vi "test4-EndNodeHandlesErrorForNotAllowedMessages.vi"(8 "error in (no error)":errorcluster, 11 "TestCase in":refnum<class "testcase-CSMChainMode.lvclass">) -> (0 "error out":errorcluster, 3 "TestCase out":refnum<class "testcase-CSMChainMode.lvclass">)   [LabVIEW 2017, in "testcase-CSMChainMode.lvclass"]
uses:
  testcase-CSMChainMode.lvclass
  src/user.lib/_NEVSTOP/Communicable State Machine(CSM)/_Support/Typedef/_CSM_MODE.ctl
  8deca385-1376-47bb-b92d-c44567c1a462.vi
  <vilib>/addons/_JKI Toolkits/VI Tester/TestCase.llb/TestCase.lvclass
  src/user.lib/_NEVSTOP/Communicable State Machine(CSM)/Communicable State Machine.lvlib
  CSM/CSM-Testcase.lvlib
  C:/Program Files (x86)/National Instruments/LabVIEW 2017/vi.lib/addons/_JKI Toolkits/VI Tester/TestCase.llb/TestCase.lvclass
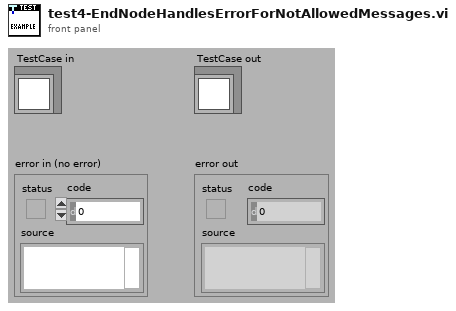
[diagram p1: front panel]
types:
  T1 = typedef "Communicable State Machine.lvlib/_CSM_MODE.ctl" = enum16{"Not Exist", "Stand Alone", "CSM", "Worker", "Worker Agent", "Chain Node", "Chain"}
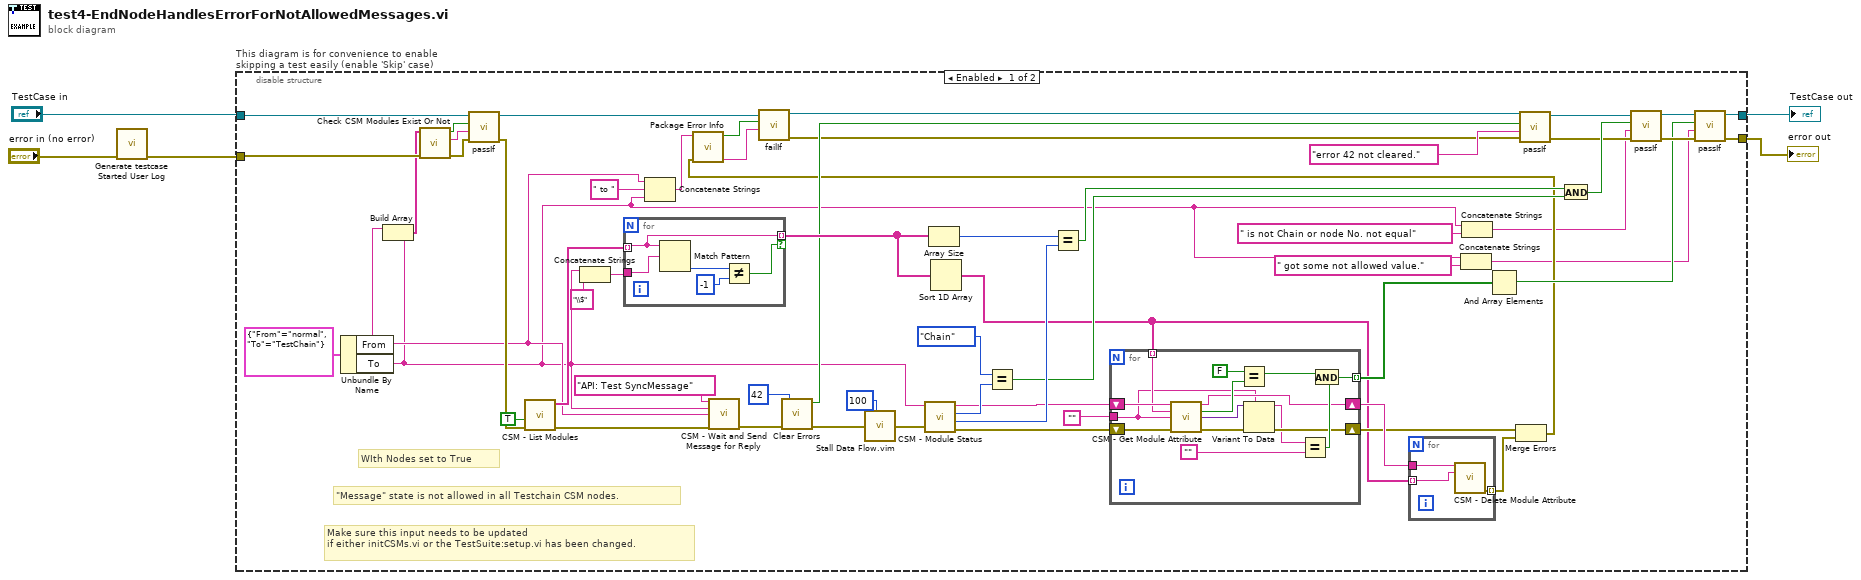
[diagram p0: block diagram]
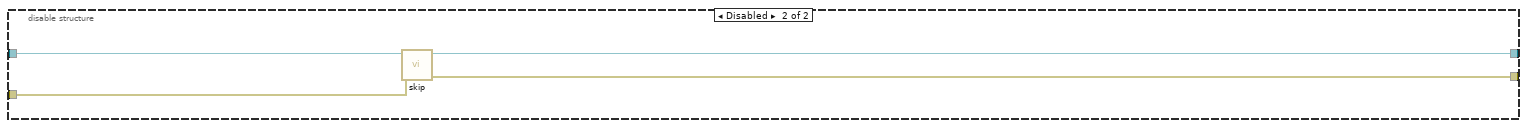
[diagram p2: hidden frame]
diagram:
  n1 = call "Generate testcase Started User Log.vi"("Error In"="error in (no error)") -> ("error out"=w1:errorcluster)  [unwired: 10 in]
  n2 = disable-structure "This diagram is for convenience to enable skipping a test easily (enable 'Skip' case)" shown="Enabled" {
    disable-tunnel: "TestCase in" -> [w19 w90]
    disable-tunnel: [w48 w88] -> w2
    disable-tunnel: [w47 w89] -> w4
    disable-tunnel: w1 -> [w17 w87]
    frame Enabled {
      # "\"Message\" state is not allowed in all Testchain CSM nodes."
      # "Make sure this input needs to be updated \nif either initCSMs.vi or the TestSuite:setup.vi has been changed."
      # "WIth Nodes set to True"
      n3 = Unbundle By Name(cluster{"From":string, "To":string} {"From"="normal", "To"="TestChain"} ("Cluster")) -> ("From"=w11:string, "To"=w8:string)
      n4 = Build Array(w11, w8) -> (w16:string[])
      n5 = call "Check CSM Modules Exist Or Not.vi"("error in"=w17, "CSM names in"=w16) -> ("error out"=w25:errorcluster, "Debug string"=w26:string, "All Modules Exist?"=w27:bool)  [unwired: 7 in]
      n6 = call-dynamic "passIf.vi"("error in (no error)"=w25, "message (\"\")"=w26, "pass"=w27, "TestCase in"=w19) -> ("error out"=w15:errorcluster, "TestCase out"=w20:refnum<class "testcase-CSMChainMode.lvclass">)  [unwired: 6 in]
      n7 = call "CSM - List Modules.vi"("Error In"=w15, "With Nodes? (F)"=TRUE) -> ("error out"=w56:errorcluster, "Module Names"=w59:string[])  [unwired: 8 in]
      n8 = Concatenate Strings(w8, "\\$" ("string")) -> (w45:string)
      n9 = for {
        tunnel: w59 -> [w84] mode=indexing
        tunnel: [w84] -> w42 mode=indexing if=w83
        tunnel: w45 -> [w82]
        n10 = Match Pattern(string=w84, regular expression=w82) -> (offset past match=w86:i32)  [unwired: 1 in, 3 out]
        n11 = Not Equal?(x=w86, y=-1) -> (x != y?=w83:bool)
      }
      n12 = Concatenate Strings(w11, " to " ("string"), w8) -> (w21:string)
      n13 = call "CSM - Wait and Send Message for Reply.vi"("State"="API: Test SyncMessage", "Arguments (\"\")"=w8, "Target Module"=w11, "Error In (No Error)"=w56) -> ("error out"=w36:errorcluster)  [unwired: 8 in, 3 out]
      n14 = call <vilib>:"Clear Errors.vi"("error in (no error)"=w36, "specific error code to clear (0: all)"=42) -> ("error out"=w39:errorcluster, "specific error cleared?"=w28:bool)  [unwired: 4 in]
      n15 = call "Stall Data Flow.vim"("value in"=w39, "milliseconds to wait"=u32 100) -> ("value out"=w61:errorcluster)  [unwired: 1 out]
      n16 = call "CSM - Module Status.vi"("Error In"=w61, "CSM Name"=w8) -> ("error out"=w38:errorcluster, "#Nodes"=w55:i32, "Mode"=w57:T1, "CSM Name (Dup)"=w37:string)  [unwired: 5 in, 1 out]
      n17 = Array Size(array=w42) -> (size(s)=w41:i32)
      n18 = Sort 1D Array(array=w42) -> (sorted array=w32:string[])
      n19 = Equal?(x=_CSM_MODE."Chain" ("Mode 2"), y=w57) -> (x = y?=w53:bool)
      n20 = Equal?(x=w41, y=w55) -> (x = y?=w54:bool)
      n21 = for {
        shift-right: [w71] -> w43
        shift-left: w37 -> [w77]
        shift-right: [w72] -> w33
        shift-left: w38 -> [w75]
        tunnel: "" -> [w68]
        tunnel: w32 -> [w76] mode=indexing
        tunnel: [w78] -> w40 mode=indexing
        n22 = call "CSM - Get Module Attribute.vi"("CSM Name"=w77, "Attribute"=w76, "Default Value (Empty Variant)"=w68, "Error In"=w75) -> ("CSM Name (Dup)"=w71:string, "Found"=w74:bool, "Value"=w70:variant, "error out"=w73:errorcluster)  [unwired: 7 in, 1 out]
        n23 = Equal?(x=FALSE, y=w74) -> (x = y?=w80:bool)
        n24 = Variant To Data(error in=w73, type=w68, Variant=w70) -> (data=w67:string, error out=w72:errorcluster)
        n25 = Equal?(x=w67, y="") -> (x = y?=w79:bool)
        n26 = And(x=w80, y=w79) -> (x .and. y?=w78:bool)
      }
      n27 = for {
        tunnel: [w66] -> w49 mode=indexing
        tunnel: w43 -> [w65]
        tunnel: w32 -> [w64] mode=indexing
        n28 = call "CSM - Delete Module Attribute.vi"("CSM Name"=w65, "Attribute"=w64) -> ("error out"=w66:errorcluster)  [unwired: 10 in, 3 out]
      }
      n29 = Concatenate Strings(w8, " got some not allowed value." ("string")) -> (w6:string)
      n30 = Concatenate Strings(w8, " is not Chain or node No. not equal" ("string")) -> (w10:string)
      n31 = And Array Elements(Boolean array=w40) -> (logical AND=w34:bool)
      n32 = Merge Errors(w33, w49) -> (w13:errorcluster)
      n33 = call "Package Error Info.vi"("error in"=w13, "String in"=w21) -> ("packed error info out"=w23:string, "error status"=w24:bool)  [unwired: 8 in]
      n34 = call-dynamic "failIf.vi"("message (\"\")"=w23, "fail"=w24, "TestCase in"=w20) -> ("error out"=w12:errorcluster, "TestCase out"=w18:refnum<class "testcase-CSMChainMode.lvclass">)  [unwired: 7 in]
      n35 = call-dynamic "passIf.vi"("error in (no error)"=w12, "message (\"\")"="error 42 not cleared." ("message (\"\")"), "pass"=w28, "TestCase in"=w18) -> ("error out"=w29:errorcluster, "TestCase out"=w30:refnum<class "testcase-CSMChainMode.lvclass">)  [unwired: 6 in]
      n36 = And(x=w54, y=w53) -> (x .and. y?=w52:bool)
      n37 = call-dynamic "passIf.vi"("error in (no error)"=w29, "message (\"\")"=w10, "pass"=w52, "TestCase in"=w30) -> ("error out"=w50:errorcluster, "TestCase out"=w51:refnum<class "testcase-CSMChainMode.lvclass">)  [unwired: 6 in]
      n38 = call-dynamic "passIf.vi"("error in (no error)"=w50, "message (\"\")"=w6, "pass"=w34, "TestCase in"=w51) -> ("error out"=w47:errorcluster, "TestCase out"=w48:refnum<class "testcase-CSMChainMode.lvclass">)  [unwired: 6 in]
    }
    frame Disabled {
      # "skip test result while test is under development"
      n39 = call <vilib>:"skip.vi"("error in (no error)"=w87, "TestCase in"=w90) -> ("error out"=w89:errorcluster, "TestCase out"=w88:refnum<class "testcase-CSMChainMode.lvclass">)  [unwired: 8 in]
    }
  }
  "error out" <- w4
  "TestCase out" <- w2
